vi "Stream Split Character Match RegExp Std Out.vi"(8 "error in (no error)":errorcluster, 11 "Example Configuration in":refnum<class "Example Custom Regex.lvclass">) -> (0 "error out":errorcluster, 2 "Stream Split Character Match RegExp Std Out":string)   [LabVIEW 2020, in "example.lvlib" / "Example Custom Regex.lvclass"]
uses:
  Example Custom Regex.lvclass
  Example Custom Regex.lvclass/Example Custom Regex.ctl
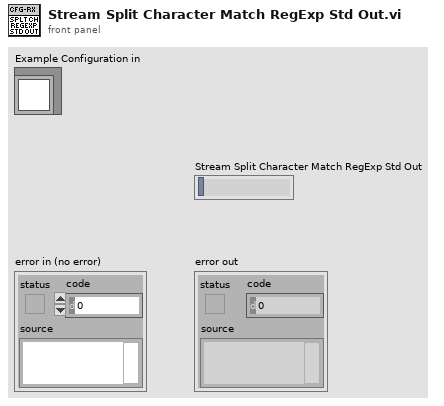
[diagram p1: front panel]
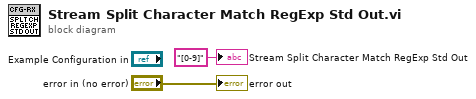
[diagram p0: block diagram]
diagram:
  "error out" <- "error in (no error)"
  "Stream Split Character Match RegExp Std Out" <- "[0-9]" ("Stream Split Character Match RegExp Std Out")
